vi "Fetch I32 data.vi"(4 "error in (no error)":errorcluster, 7 "Statement Refnum":T1) -> (0 "error out":errorcluster, 2 "Data":i32, 3 "Statement Refnum":T1)   [LabVIEW 2011]
doc: "Lit la donnée de type entier long (I32)"
uses:
  SQL Controls/Statement Refnum.ctl
  Odbc32.dll
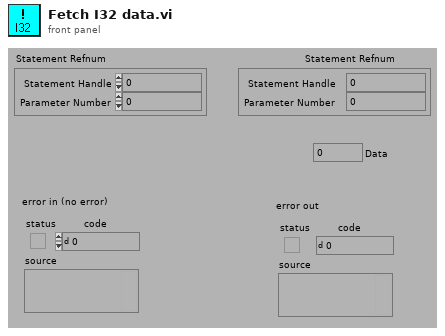
[diagram p1: front panel]
types:
  T1 = typedef "Statement Refnum.ctl" = cluster{"Statement Handle":i32, "Parameter Number":u16}
  T2 = enum16{"NOPE", "SQL_HANDLE_ENV", "SQL_HANDLE_DBC", "SQL_HANDLE_STMT", "SQL_HANDLE_DESC"}
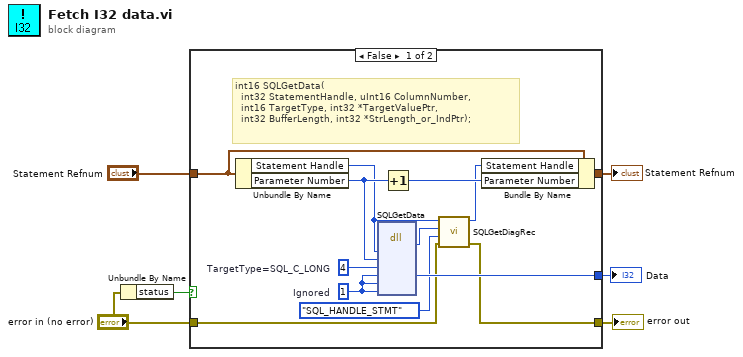
[diagram p0: block diagram]
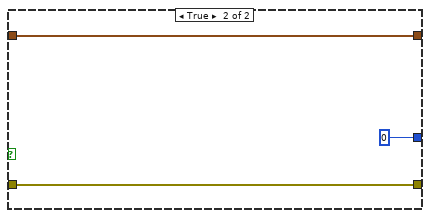
[diagram p2: hidden frame]
diagram:
  n1 = Unbundle By Name("error in (no error)") -> ("status"=w1:bool)
  n2 = case shown="False" w1 {
    tunnel: [w19 0] -> w6
    tunnel: "Statement Refnum" -> [w18 w20]
    tunnel: [w17 w20] -> w4
    tunnel: "error in (no error)" -> [w9 w22]
    tunnel: [w8 w22] -> w2
    frame False {
      w13 = i16 4  # TargetType=SQL_C_LONG
      w14 = 1  # Ignored
      # "int16 SQLGetData(\n  int32 StatementHandle, uInt16 ColumnNumber, \n  int16 TargetType, int32 *TargetValuePtr,\n  int32 BufferLength, int32 *StrLength_or_IndPtr);"
      n3 = Unbundle By Name(w18) -> ("Statement Handle"=w12:i32, "Parameter Number"=w16:u16)
      n4 = dll-call lib="Odbc32.dll" fn="SQLGetData"("StatementHandle"=w12, "ColumnNumber"=w16, "TargetType"=w13, "TargetValuePtr"=w14, "BufferLength"=w14, "StrLength_or_IndPtr"=w14) -> (w11:i16, "TargetValuePtr"=w19:i32)  [unwired: 7 in, 3 out]
      n5 = Increment(x=w16) -> (x+1=w15:u16)
      n6 = call "SQLGetDiagRec.vi"("error in (no error)"=w9, "HandleType"=T2."SQL_HANDLE_STMT", "Status (SQL_SUCCESS=0)"=w11, "Input Handle"=w12) -> ("error out"=w8:errorcluster, "Output Handle"=w10:i32)  [unwired: 2 out]
      n7 = Bundle By Name(cluster=w18, "Statement Handle"=w10, "Parameter Number"=w15) -> (w17:T1)
    }
    frame True {
    }
  }
  "Statement Refnum" <- w4
  "Data" <- w6
  "error out" <- w2
